vi "Write.vi"(8 "error in (no error)":errorcluster, 10 "Boolean":T1, 11 "Local Bus_DBL in":refnum<class "Fault-Injection_Boolean.lvclass">) -> (0 "error out":errorcluster, 3 "Local Bus_DBL out":refnum<class "Fault-Injection_Boolean.lvclass">)   [LabVIEW 2021, in "Fault-Injection_Boolean.lvclass"]
uses:
  Fault-Injection_Boolean.lvclass
  Support/Value Type.ctl
  Fault-Injection_Boolean.lvclass/Fault-Injection_Boolean.ctl
  <vilib>/TSA/Abstract Data Classes/Abs_Types/Boolean/Abs_Boolean.lvclass
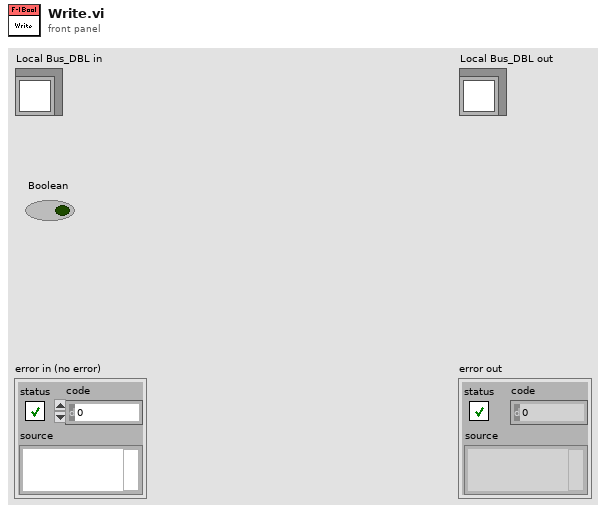
[diagram p1: front panel]
types:
  T1 = typedef "Fault-Injection_Boolean.lvclass/Value Type.ctl" = bool
  T2 = typedef "Fault-Injection_Boolean.lvclass/DVR Type.ctl" = cluster{"Enable":bool, "Injected Value":T1, "Value":refnum<class "Abs_Boolean.lvclass">}
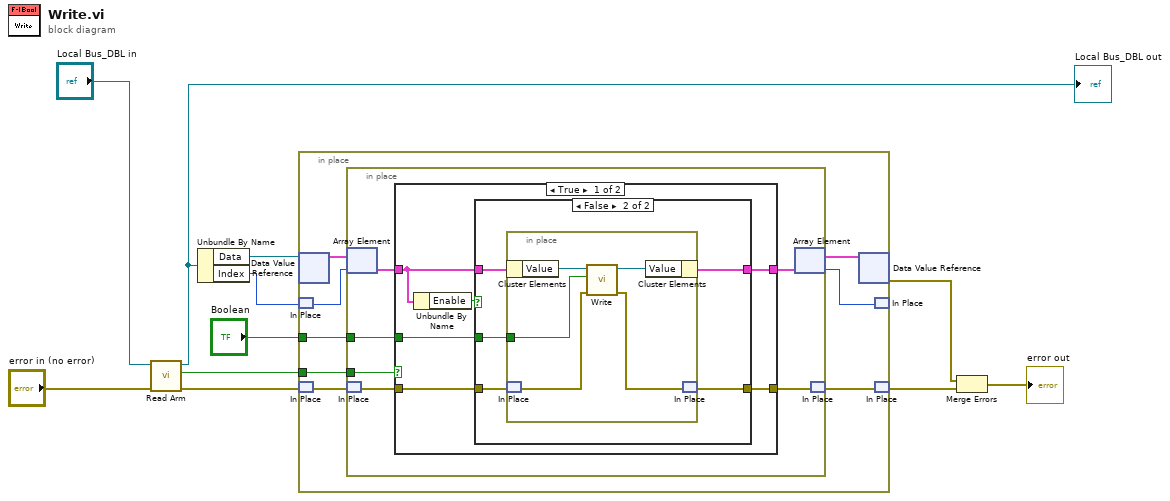
[diagram p0: block diagram]
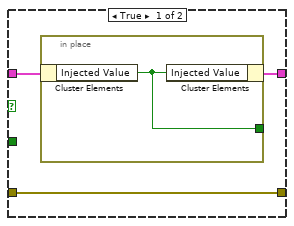
[diagram p2: hidden frame]
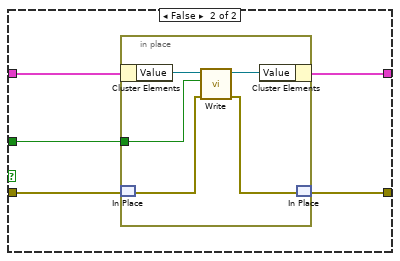
[diagram p3: hidden frame]
diagram:
  n1 = call-dynamic "Read Arm.vi"("error in (no error)"="error in (no error)", "Fault-Injection_Boolean in"="Local Bus_DBL in") -> ("error out"=w7:errorcluster, "Armed?"=w6:bool, "Fault-Injection_Boolean out"=w5:refnum<class "Fault-Injection_Boolean.lvclass">)  [unwired: 7 in]
  "Local Bus_DBL out" <- w5
  n2 = Unbundle By Name(w5) -> ("Data"=w11:refnum<data-value>, "Index"=w10:i32)
  n3 = in-place {
    in-place-border: w6 -> [w13]
    in-place-border: "Boolean" -> [w12]
    n4 = in-place-dvr #1(w11) -> (w19:T2[])  [unwired: 1 out]
    n5 = in-place-match #2(w10) -> (w17:i32)
    n6 = in-place-match #3(w7) -> (w15:errorcluster)
    n7 = in-place {
      in-place-border: w13 -> [w21]
      in-place-border: w12 -> [w20]
      n8 = in-place-array #4(w19, w17) -> (w22:T2)
      n9 = in-place-match #5(w15) -> (w24:errorcluster)
      n10 = case shown="True" w21 {
        tunnel: [w31 w50] -> w25
        tunnel: w24 -> [w30 w49]
        tunnel: [w29 w48] -> w23
        tunnel: w22 -> [w27 w47]
        tunnel: w20 -> [w26 w46]
        frame True {
          n11 = Unbundle By Name(w27) -> ("Enable"=w28:bool)
          n12 = case shown="False" w28 {
            tunnel: w27 -> [w34 w40]
            tunnel: [w33 w39] -> w31
            tunnel: w30 -> [w32 w38]
            tunnel: [w32 w37] -> w29
            tunnel: w26 -> [_ w36]
            frame True {
              n13 = in-place {
                in-place-border: [w35] -> _
                n14 = in-place-cluster #6(w34) -> ("Injected Value"=w35:T1)
                n15 = in-place-cluster #6("Injected Value"=w35) -> (w33:T2)
              }
            }
            frame False {
              n16 = in-place {
                in-place-border: w36 -> [w41]
                n17 = in-place-cluster #7(w40) -> ("Value"=w42:refnum<class "Abs_Boolean.lvclass">)
                n18 = in-place-match #8(w38) -> (w44:errorcluster)
                n19 = call-dynamic "Write.vi"("error in (no error)"=w44, "Boolean"=w41, "Boolean in"=w42) -> ("error out"=w43:errorcluster, "Boolean out"=w45:refnum<class "Abs_Boolean.lvclass">)  [unwired: 7 in]
                n20 = in-place-cluster #7("Value"=w45) -> (w39:T2)
                n21 = in-place-match #8(w43) -> (w37:errorcluster)
              }
            }
          }
        }
        frame False {
          n22 = in-place {
            in-place-border: w46 -> [w51]
            n23 = in-place-cluster #9(w47) -> ("Value"=w54:refnum<class "Abs_Boolean.lvclass">)
            n24 = in-place-match #10(w49) -> (w53:errorcluster)
            n25 = call-dynamic "Write.vi"("error in (no error)"=w53, "Boolean"=w51, "Boolean in"=w54) -> ("error out"=w52:errorcluster, "Boolean out"=w55:refnum<class "Abs_Boolean.lvclass">)  [unwired: 7 in]
            n26 = in-place-cluster #9("Value"=w55) -> (w50:T2)
            n27 = in-place-match #10(w52) -> (w48:errorcluster)
          }
        }
      }
      n28 = in-place-array #4(w25) -> (w18:T2[], w16:i32)
      n29 = in-place-match #5(w23) -> (w14:errorcluster)
    }
    n30 = in-place-dvr #1(w18) -> (w8:errorcluster)  [unwired: 1 out]
    n31 = in-place-match #2(w16) -> ()  [unwired: 1 out]
    n32 = in-place-match #3(w14) -> (w9:errorcluster)
  }
  n33 = Merge Errors(w8, w9) -> (→"error out":errorcluster)
